vi "Operadores Logicos.vi"() -> ()   [LabVIEW 2015]
panel:
  out "Xnor":bool
  out "Nor":bool
  out "Nand":bool
  out "Xor":bool
  out "Or":bool
  out "And":bool
  out "Boolean":bool
  in  "B":bool
  in  "A":bool
  in  "Not":bool
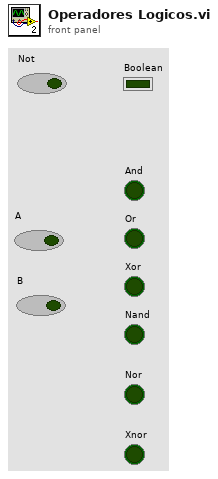
[diagram p1: front panel]
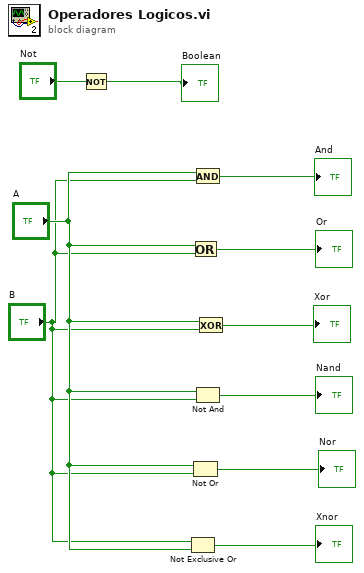
[diagram p0: block diagram]
diagram:
  n1 = Not(x="Not") -> (.not. x?=→"Boolean":bool)
  n2 = Not Exclusive Or(1:"A", 2:"B") -> (0:→"Xnor":bool)
  n3 = Not Or(1:"B", 2:"A") -> (0:→"Nor":bool)
  n4 = Or(x="A", y="B") -> (x .or. y?=→"Or":bool)
  n5 = And(x="A", y="B") -> (x .and. y?=→"And":bool)
  n6 = Not And(1:"B", 2:"A") -> (0:→"Nand":bool)
  n7 = Exclusive Or(1:"B", 2:"A") -> (0:→"Xor":bool)
